vi "Read Status Byte Query.vi"(0 "VISA resource name":refnum<visa-resource-name>, 11 "error in (no error)":errorcluster) -> (4 "VISA resource name out":refnum<visa-resource-name>, 6 "Status Byte Register":T1, 15 "error out":errorcluster)   [LabVIEW 2020, in "NH Research Regenerative Test Series.lvlib"]
doc: "Queries the <B>Status Byte</B>. Returns the decimal value of the binary-weighted sum of bits.\n\nEach bit represents a status in the instrument.\n\nEx : When the module is busy, Bit 0 is set High giving status \"Module is Busy\"\n\nBit 0: Module is Busy\nBit 1: Module in Remote Mode\nBit 2: Error in Queue\nBit 3: QUES = Questionable Status Summary\nBit 4: MAV = Message Available\nBit 5: ESB = Event Status Byte Summary\nBit 6: RQS = Request for Service\nBit 7: OPER = Operation Event Summary"
uses:
  NH Research Regenerative Test Series.lvlib
panel:
  # "Bit 0: Module is Busy\nBit 1: Module in Remote Mode\nBit 2: Error in Queue\nBit 3: QUES = Questionable Status Summary\nBit 4: MAV = Message Available\nBit 5: ESB = Event Status Byte Summary\nBit 6: RQS = Request for Service\nBit 7: OPER = Operation Event Summary"
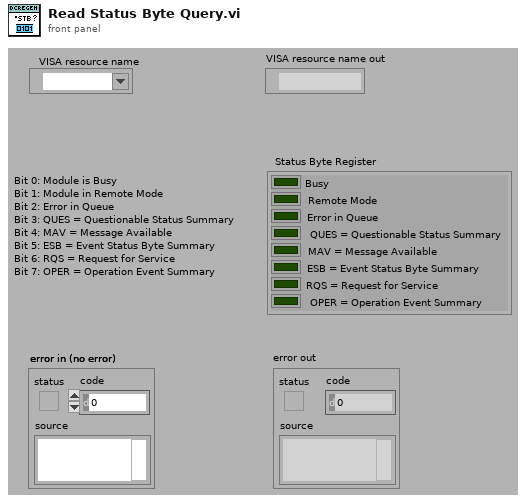
[diagram p1: front panel]
types:
  T1 = cluster{"Busy":bool, "Remote Mode":bool, "Error in Queue":bool, "QUES = Questionable Status Summary":bool, "MAV = Message Available":bool, "ESB = Event Status Byte Summary":bool, "RQS = Request for Service":bool, "OPER = Operation Event Summary":bool}
  T2 = cluster{"Boolean array[0]":bool, "Boolean array[1]":bool, "Boolean array[2]":bool, "Boolean array[3]":bool, "Boolean array[4]":bool, "Boolean array[5]":bool, "Boolean array[6]":bool, "Boolean array[7]":bool}
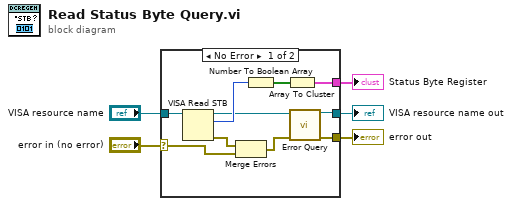
[diagram p0: block diagram]
diagram:
  n1 = case shown="No Error" "error in (no error)" {
    selector: "error in (no error)" -> [w6 w16]
    tunnel: [w15 _] -> w5
    tunnel: "VISA resource name" -> [w14 w17]
    tunnel: [w13 w17] -> w3
    tunnel: [w12 w16] -> w2
    frame No Error {
      n2 = VISA Read STB(11:w14) -> (0:w8:errorcluster, 2:w11:u16, 3:w9:refnum<visa-resource-name>)  [unwired: 1 in]
      n3 = Merge Errors(w8, w6) -> (w7:errorcluster)
      n4 = Number To Boolean Array(number=w11) -> (Boolean array=w10:bool[])
      n5 = Array To Cluster(array=w10) -> (cluster=w15:T2)
      n6 = call "Error Query.vi"("VISA resource name"=w9, "error in (no error)"=w7) -> ("VISA resource name out"=w13:refnum<visa-resource-name>, "error out"=w12:errorcluster)  [unwired: 10 in, 2 out]
    }
    frame Error {
    }
  }
  "Status Byte Register" <- w5
  "VISA resource name out" <- w3
  "error out" <- w2
